vi "Uninit_library.vi"(8 "error in":errorcluster) -> (0 "error out":errorcluster)   [LabVIEW 2019, in "PICam.lvlib"]
doc: "Picam_UninitializeLibrary() frees resources that have been used by the API Library,\nincluding open cameras and memory."
uses:
  PICam.lvlib
  Picam64.dll   
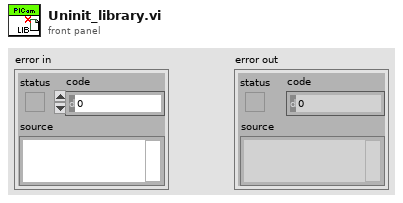
[diagram p1: front panel]
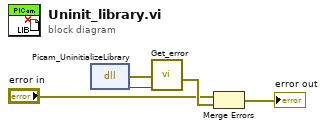
[diagram p0: block diagram]
diagram:
  n1 = dll-call lib="Picam32.dll" fn="Picam_UninitializeLibrary"() -> (error out=w5:errorcluster, "return type"=w4:i32)  [unwired: 3 in, 1 out]
  n2 = call "Get_error.vi"("PICam_Error"=w4, "error in (no error)"=w5) -> ("error out"=w2:errorcluster)  [unwired: 9 in]
  n3 = Merge Errors("error in", w2) -> (→"error out":errorcluster)
